vi "create request byte.vi"(11 "x":u32) -> (1 "output array 2":u8[](array[numeric]) format="%.0x", 3 "output array":u8[](array[numeric]) format="%.0x")   [LabVIEW 2014]
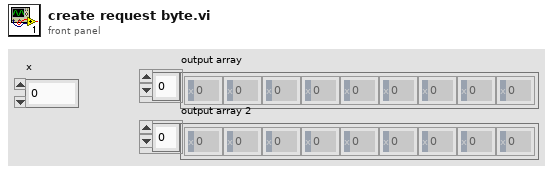
[diagram p1: front panel]
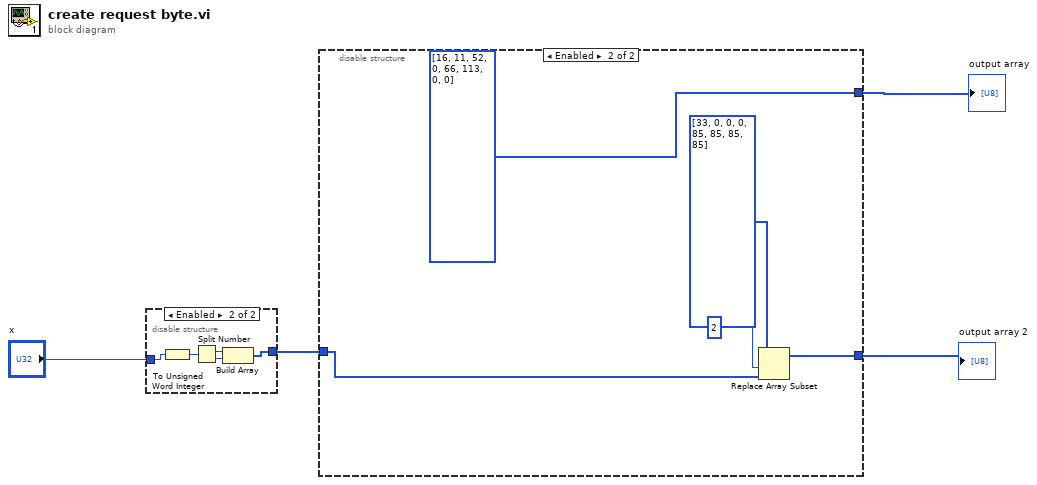
[diagram p0: block diagram]
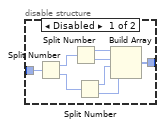
[diagram p2: hidden frame]
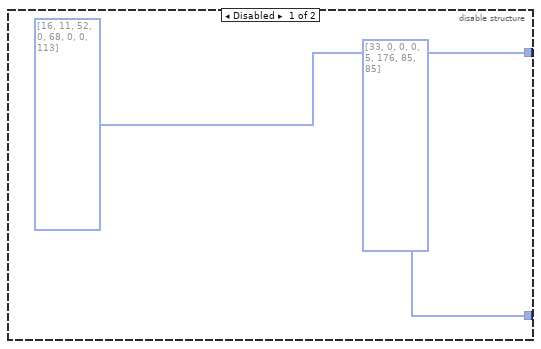
[diagram p3: hidden frame]
diagram:
  n1 = disable-structure shown="Enabled" {
    disable-tunnel: [w12 w13] -> w4
    disable-tunnel: "x" -> [w5 w14]
    frame Disabled {
      n2 = Split Number(x=w5) -> (hi(x)=w10:u16, lo(x)=w11:u16)
      n3 = Split Number(x=w10) -> (hi(x)=w9:u8, lo(x)=w8:u8)
      n4 = Split Number(x=w11) -> (hi(x)=w7:u8, lo(x)=w6:u8)
      n5 = Build Array(w9, w8, w7, w6) -> (w12:u8[])
    }
    frame Enabled {
      n6 = To Unsigned Word Integer(number=w14) -> (unsigned 16bit integer=w17:u16)
      n7 = Split Number(x=w17) -> (hi(x)=w16:u8, lo(x)=w15:u8)
      n8 = Build Array(w16, w15) -> (w13:u8[])
    }
  }
  n9 = disable-structure shown="Enabled" {
    disable-tunnel: w4 -> [_ w21]
    disable-tunnel: [u8[] [33, 0, 0, 0, 5, 176, 85, 85] ("payload") w22] -> w3
    disable-tunnel: [u8[] [16, 11, 52, 0, 68, 0, 0, 113] ("payload") u8[] [16, 11, 52, 0, 66, 113, 0, 0] ("payload")] -> w1
    frame Disabled {
    }
    frame Enabled {
      n10 = Replace Array Subset(array=u8[] [33, 0, 0, 0, 85, 85, 85, 85] ("payload"), new element=w21, index=2) -> (w22:u8[])
    }
  }
  "output array 2" <- w3
  "output array" <- w1
